vi "Burst.vi"(0 "RFFE RegReadExt Command in":refnum<class "RFFE RegReadExt Command.lvclass">, 1 "Bus Number":i32, 5 "instrument handle in":refnum<k15>, 11 "error in (no error)":errorcluster) -> (4 "RFFE RegReadExt Command out":refnum<class "RFFE RegReadExt Command.lvclass">, 6 "instrument handle out":refnum<k15>, 15 "error out":errorcluster)   [LabVIEW 2018, in "MIPI RFFE API.lvlib" / "RFFE RegReadExt Command.lvclass"]
uses:
  RFFE RegReadExt Command.lvclass
  C:/Users/semoore/Projects/mipi-rffe-labview-oop/Extended Command/RFFE Extended Command.lvclass
  Extended Command/RFFE Extended Command.lvclass/RFFE Extended Command.ctl
  Extended Command/Set Register Data.vi
  Extended Command/RFFE Extended Command.lvclass
  MIPI RFFE API.lvlib
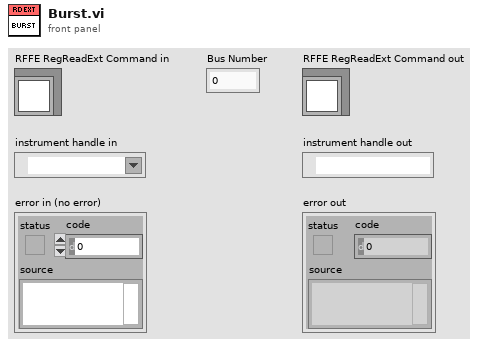
[diagram p1: front panel]
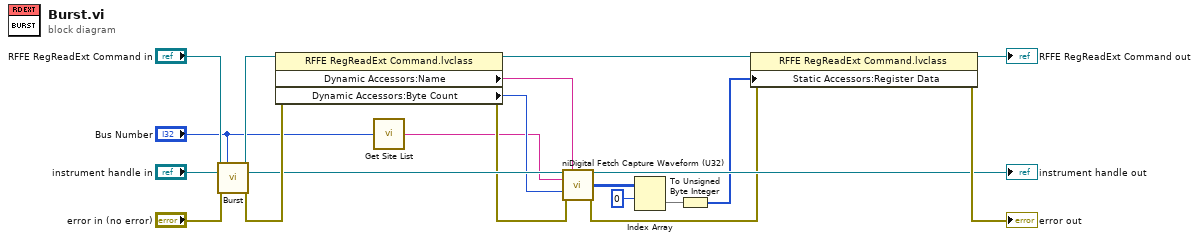
[diagram p0: block diagram]
diagram:
  n1 = call-parent "Burst.vi"("RFFE Command in"="RFFE RegReadExt Command in", "Bus Number"="Bus Number", "instrument handle in"="instrument handle in", "error in (no error)"="error in (no error)") -> ("RFFE Command out"=w19:refnum<class "RFFE RegReadExt Command.lvclass">, "instrument handle out"=w12:refnum<k15>, "error out"=w14:errorcluster)  [unwired: 9 in]
  n2 = property class="RFFE RegReadExt Command.lvclass"(reference=w19, error in=w14) -> (reference out=w8:refnum<class "RFFE RegReadExt Command.lvclass">, error out=w9:errorcluster, "Dynamic Accessors:Name"=w10:string, "Dynamic Accessors:Byte Count"=w2:i32)
  n3 = call "Get Site List.vi"("Bus Number"="Bus Number") -> ("Site List"=w1:string)  [unwired: 14 in]
  n4 = call <instrlib>:"niDigital Fetch Capture Waveform (U32).vi"("instrument handle"=w12, "waveform name"=w10, "site list"=w1, "samples to read"=w2, "error in"=w9) -> ("instrument handle out"=→"instrument handle out":refnum<k15>, "data"=w6:u32[][], "error out"=w7:errorcluster)  [unwired: 8 in]
  n5 = Index Array(array=w6, index (row)=0) -> (element=w4:u32[])  [unwired: 1 in]
  n6 = To Unsigned Byte Integer(number=w4) -> (unsigned 8bit integer=w3:u8[])
  n7 = property class="RFFE RegReadExt Command.lvclass"(reference=w8, error in=w7, "Static Accessors:Register Data"=w3) -> (reference out=→"RFFE RegReadExt Command out":refnum<class "RFFE RegReadExt Command.lvclass">, error out=→"error out":errorcluster)
